vi "Create Transport DAT File.vi"(6 "append to existing file?\n(new file:F)":bool, 8 "error in (no error)":errorcluster, 10 "Wavenames":string[](array[string]), 11 "Control Experiment in":refnum<class "AFM Control.lvclass">) -> (0 "error out":errorcluster, 3 "Control Experiment out":refnum<class "AFM Control.lvclass">)   [LabVIEW 2016]
uses:
  AFM Control.lvclass
  <userlib>/LevyLab/LV to ITX/LVtoITX.lvclass
  <userlib>/LevyLab/LV to ITX/Main/LV to DAT 1D.vi
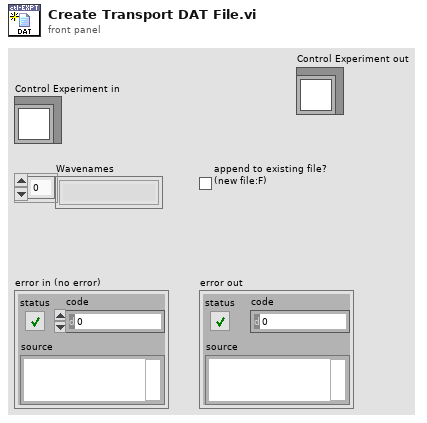
[diagram p1: front panel]
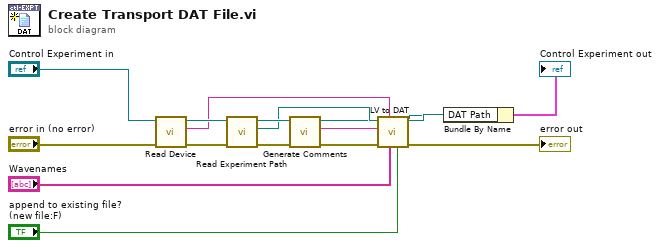
[diagram p0: block diagram]
diagram:
  n1 = call "Read Device.vi"("error in (no error)"="error in (no error)", "AFM Control"="Control Experiment in") -> ("error out"=w11:errorcluster, "Device"=w5:string, "AFM Control out"=w7:refnum<class "AFM Control.lvclass">)  [unwired: 7 in]
  n2 = call "Read Experiment Path.vi"("error in (no error)"=w11, "AFM Control"=w7) -> ("error out"=w10:errorcluster, "Experiment Path"=w4:path, "AFM Control out"=w8:refnum<class "AFM Control.lvclass">)  [unwired: 7 in]
  n3 = call "Generate Comments.vi"("error in (no error)"=w10, "AFM Control"=w8) -> ("error out"=w9:errorcluster, "Comments"=w6:string, "AFM Control out"=w2:refnum<class "AFM Control.lvclass">)  [unwired: 6 in]
  n4 = call-poly <userlib>:"LV to DAT.vi"("append to file? (new file:F)"="append to existing file?\n(new file:F)", "wavenames (.Vx, etc)"="Wavenames", "filename"=w5, "error in"=w9, "Comments"=w6, "path"=w4) -> ("error out"=→"error out":errorcluster, "new file path"=w3:path)  [unwired: 4 in]
  n5 = Bundle By Name(cluster=w2, "DAT Path"=w3) -> (→"Control Experiment out":cluster{})
